vi "random.vi"(8 "Min value":dbl, 11 "Max value":dbl) -> (0 "Sortie inv":dbl, 3 "Sortie":dbl)   [LabVIEW 2019]
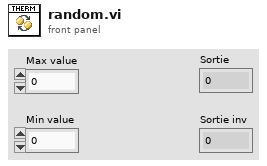
[diagram p1: front panel]
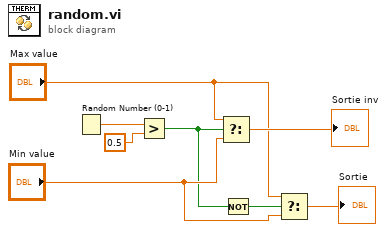
[diagram p0: block diagram]
diagram:
  n1 = Random Number (0-1)() -> (number: 0 to 1=w3:dbl)
  n2 = Greater?(x=w3, y=0.5) -> (0:w1:bool)
  n3 = Select(t="Max value", s=w1, f="Min value") -> (s? t:f=→"Sortie inv":dbl)
  n4 = Not(x=w1) -> (.not. x?=w7:bool)
  n5 = Select(t="Max value", s=w7, f="Min value") -> (s? t:f=→"Sortie":dbl)
